vi "SaveToMemory.vi"(4 "error in (no error)":errorcluster, 5 "Device Address In":i32, 6 "DeviceKey In":string, 7 "CmdLib In":refnum<k24>) -> (0 "error out":errorcluster, 1 "Device Address Out":i32, 2 "DeviceKey Out":string, 3 "CmdLib Out":refnum<k24>)   [LabVIEW 2024]
uses:
  C:/Development/Prime-RIMAS/Focus/PicoMotor/CmdLib.dll
  CmdLib.dll
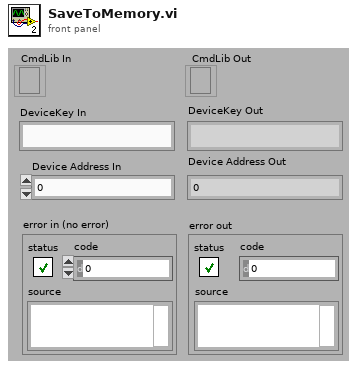
[diagram p1: front panel]
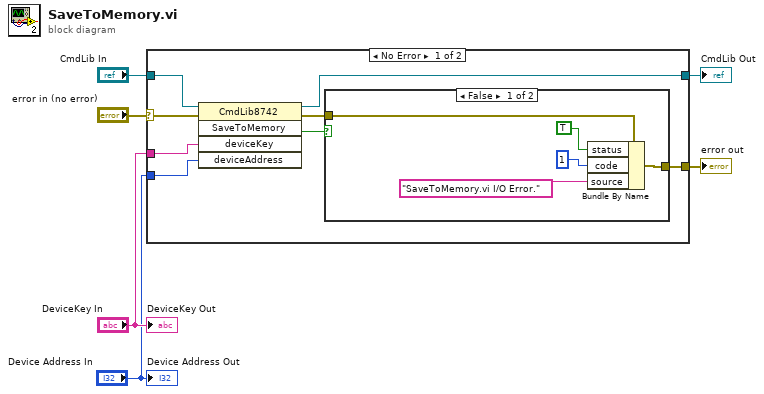
[diagram p0: block diagram]
diagram:
  n1 = case shown="No Error" "error in (no error)" {
    selector: "error in (no error)" -> [w11 w21]
    tunnel: "CmdLib In" -> [w14 w22]
    tunnel: [w13 w22] -> w5
    tunnel: "DeviceKey In" -> [w12 _]
    tunnel: [w8 w21] -> w2
    tunnel: "Device Address In" -> [w7 _]
    frame No Error {
      n2 = invoke class="CmdLib8742" method="SaveToMemory"(reference=w14, error in=w11, "deviceKey"=w12, "deviceAddress"=w7) -> (reference out=w13:refnum<k24>, error out=w9:errorcluster, "SaveToMemory"=w10:bool)  [unwired: 1 in, 2 out]
      n3 = case shown="False" w10 {
        tunnel: w9 -> [w19 w20]
        tunnel: [w18 w20] -> w8
        frame False {
          n4 = Bundle By Name(cluster=w19, "status"=TRUE, "code"=1, "source"="SaveToMemory.vi I/O Error.") -> (w18:errorcluster)
        }
        frame True {
        }
      }
    }
    frame Error {
    }
  }
  "error out" <- w2
  "CmdLib Out" <- w5
  "DeviceKey Out" <- "DeviceKey In"
  "Device Address Out" <- "Device Address In"
